vi "TestExecuteDefaultPolicy_PublishOK.vi"(8 "error in (no error)":errorcluster, 11 "TestCase in":refnum<class "TestSubscriptionPolicy.lvclass">) -> (0 "error out":errorcluster, 3 "TestCase out":refnum<class "TestSubscriptionPolicy.lvclass">)   [LabVIEW 2015, in "TestSubscriptionPolicy.lvclass"]
uses:
  TestSubscriptionPolicy.lvclass
  Framework/IMediator/ISubscriptionPolicy/ISubscriptionPolicy.lvclass
  Framework/Mediator/Transport/QueueTransport/QueueTransport.lvclass
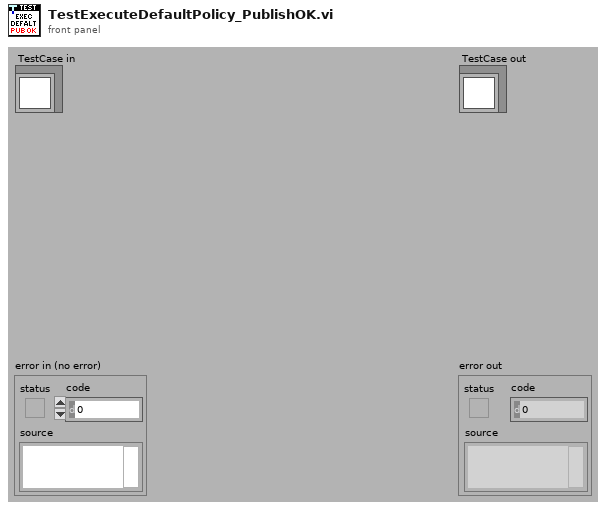
[diagram p1: front panel]
types:
  T1 = cluster{"Data":variant, "Publication Time":timestamp}
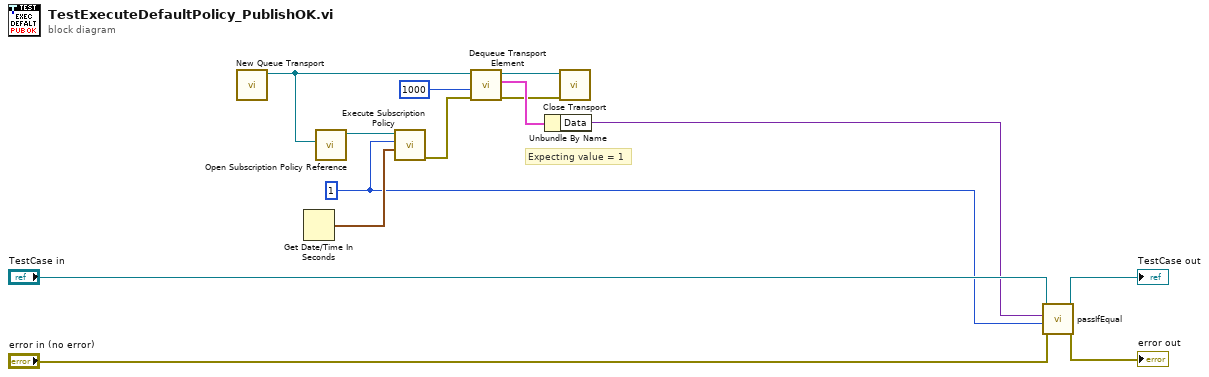
[diagram p0: block diagram]
diagram:
  w1 = 1
  # "Expecting value = 1"
  n1 = call "New Queue Transport.vi"() -> ("QueueTransport Out"=w9:refnum<class "QueueTransport.lvclass">)  [unwired: 10 in, 1 out]
  n2 = Get Date/Time In Seconds() -> (seconds since 1Jan1904=w5:timestamp)
  n3 = call "Open Subscription Policy Reference.vi"("Transport"=w9) -> ("Subscription Policy"=w10:refnum<data-value>)  [unwired: 9 in, 1 out]
  n4 = call "Execute Subscription Policy.vi"("Publish Time"=w5, "New Topic Value"=w1, "Subscription Policy"=w10) -> ("error out (Unsubscribe?)"=w8:errorcluster)  [unwired: 8 in]
  n5 = call "Dequeue Transport Element.vi"("error in (no error)"=w8, "Timeout In ms (-1)"=1000, "QueueTransport in"=w9) -> ("error out"=w3:errorcluster, "Element"=w6:T1, "QueueTransport out"=w4:refnum<class "QueueTransport.lvclass">)  [unwired: 5 in, 1 out]
  n6 = Unbundle By Name(w6) -> ("Data"=w2:variant)
  n7 = call-dynamic "Close Transport.vi"("error in (no error)"=w3, "QueueTransport in"=w4) -> ()  [unwired: 9 in, 1 out]
  n8 = call-dynamic "passIfEqual.vi"("error in (no error)"="error in (no error)", "y"=w1, "x"=w2, "TestCase in"="TestCase in") -> ("error out"=→"error out":errorcluster, "TestCase out"=→"TestCase out":refnum<class "TestSubscriptionPolicy.lvclass">)  [unwired: 6 in]
